vi "Undo.vi"(0 "reference in":refnum<class "SpindleOnCommand.lvclass">, 5 "error in (no error)":errorcluster) -> (14 "reference out":refnum<class "SpindleOnCommand.lvclass">, 19 "error out":errorcluster)   [LabVIEW 2013, in "SpindleOnCommand.lvclass"]
uses:
  SpindleOnCommand.lvclass
  Spindle_class/Spindle.lvclass
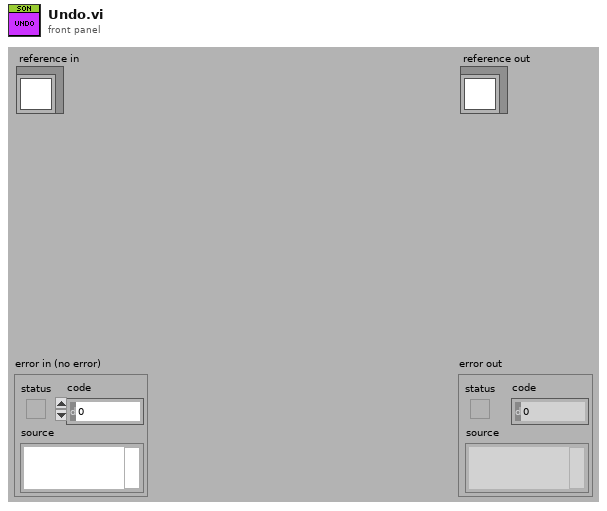
[diagram p1: front panel]
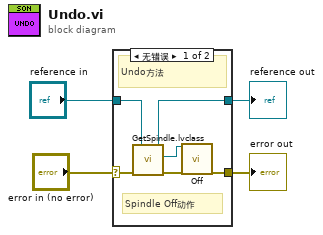
[diagram p0: block diagram]
diagram:
  n1 = case shown="无错误" "error in (no error)" {
    selector: "error in (no error)" -> [w7 w12]
    tunnel: [w5 w12] -> w3
    tunnel: [w9 w11] -> w1
    tunnel: "reference in" -> [w10 w11]
    frame No Error {
      # "Spindle Off动作"
      # "Undo方法"
      n2 = call-dynamic "GetSpindle.lvclass.vi"("error in (no error)"=w7, "reference in"=w10) -> ("error out"=w6:errorcluster, "Spindle.lvclass"=w8:refnum<class "Spindle.lvclass">, "reference out"=w9:refnum<class "SpindleOnCommand.lvclass">)  [unwired: 7 in]
      n3 = call-dynamic "Off.vi"("reference in"=w8, "error in (no error)"=w6) -> ("error out"=w5:errorcluster)  [unwired: 16 in, 1 out]
    }
    frame Error {
    }
  }
  "error out" <- w3
  "reference out" <- w1
